vi "Log File Inspector.vi"(1 "Thermocouple types":T4[](array[typedef])=[3, 3, 3, 3, 3, 3, 3, 3, 3, 3, 6, 6, 6, 6, 6, 6] items=["B", "E", "J", "K", "R", "S", "T", "N"], 2 "LC Calibration":T2, 3 "PS Calibration":T3) -> ()   [LabVIEW 2017]
uses:
  Controls/LC Calibration Cluster.ctl
  Support Vis/HOST/cRIO Convert Thermocouple Readings.llb/Thermocouple Type.ctl
  Controls/PS Calibration Cluster.ctl
panel:
  in  "Settings Tab 3":T1(tab)
  out "Temperature Graph":cluster{dbl[], "Y":dbl[]}[](graph)
  out "Pressure Graph":cluster{dbl[], "Y":dbl[]}[](graph)
  out "Load Cell Graph":cluster{dbl[], "Y":dbl[]}[](graph)
  out "Valve Graph":cluster{dbl[], "Y":dbl[]}[](graph)
  in  "Stop Button":bool
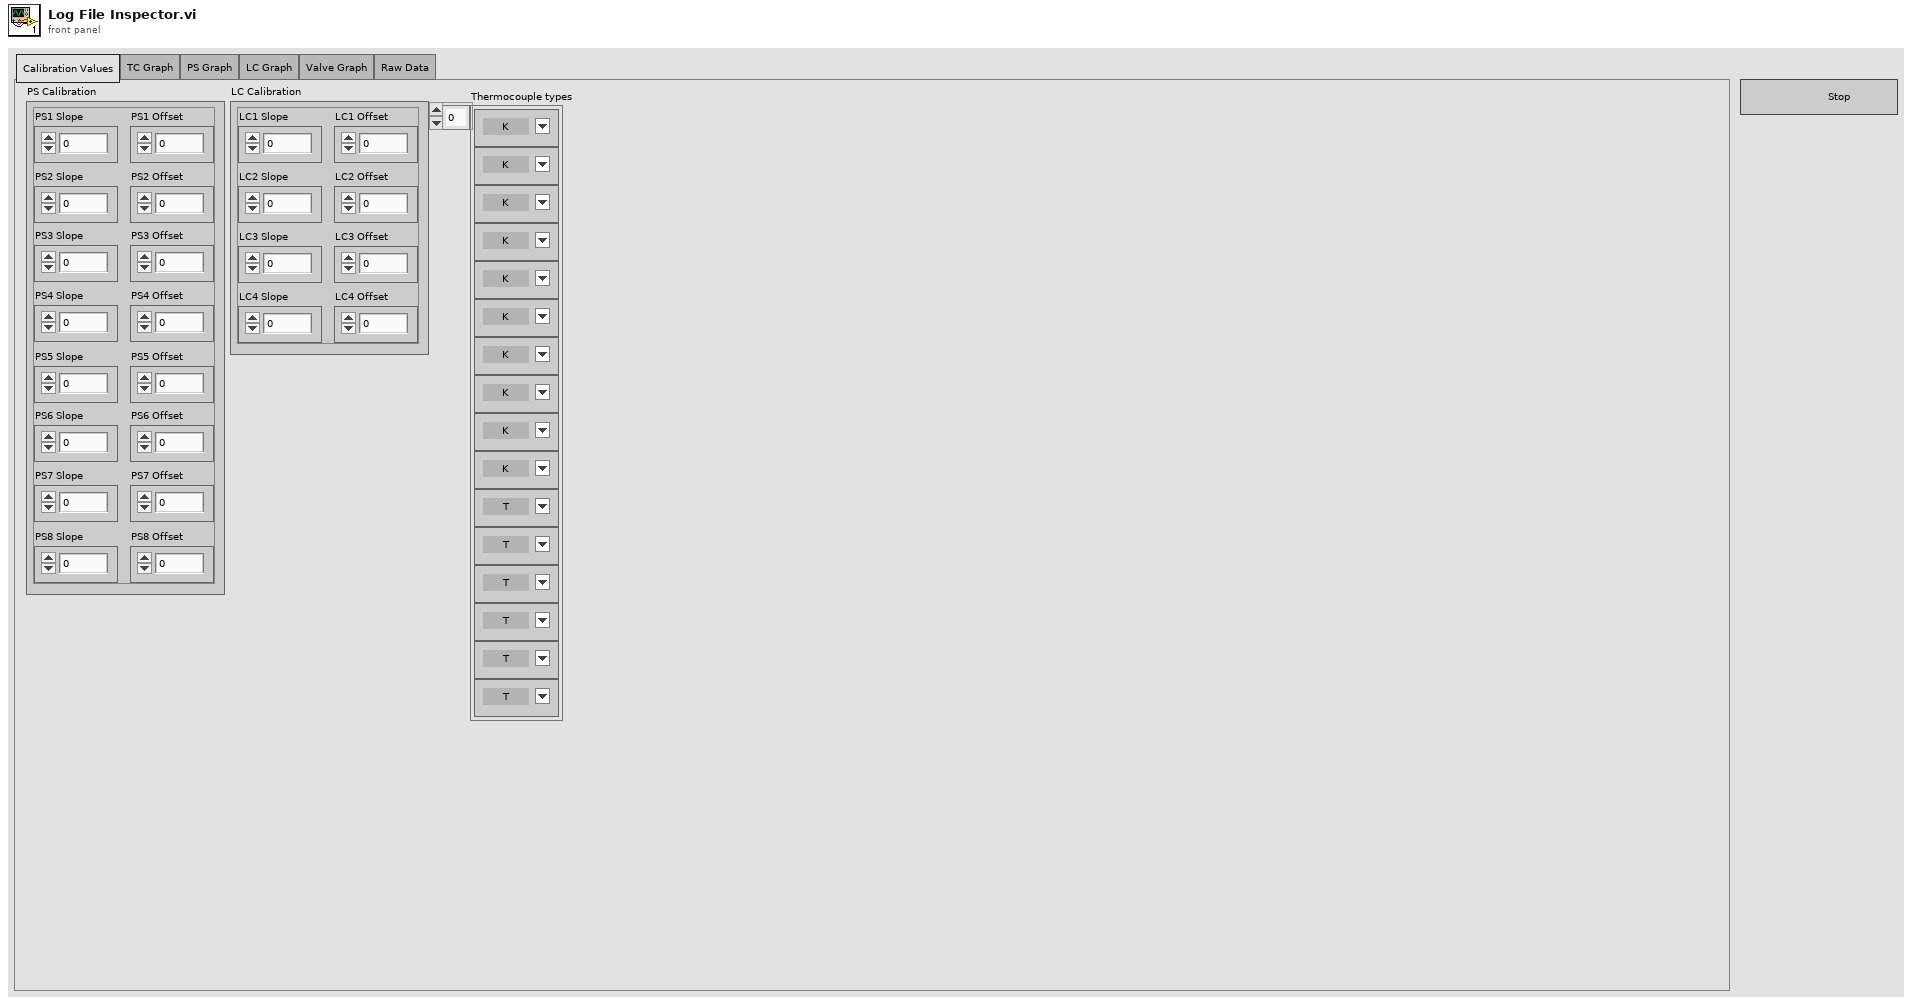
[diagram p1: front panel]
types:
  T1 = enum32{"Calibration Values", "TC Graph", "PS Graph", "LC Graph", "Valve Graph", "Raw Data"}
  T2 = typedef "LC Calibration Cluster.ctl" = cluster{"LC1 Slope":dbl, "LC1 Offset":dbl, "LC2 Slope":dbl, "LC2 Offset":dbl, "LC3 Slope":dbl, "LC3 Offset":dbl, "LC4 Slope":dbl, "LC4 Offset":dbl}
  T3 = typedef "PS Calibration Cluster.ctl" = cluster{"PS1 Slope":dbl, "PS1 Offset":dbl, "PS2 Slope":dbl, "PS2 Offset":dbl, "PS3 Slope":dbl, "PS3 Offset":dbl, "PS4 Slope":dbl, "PS4 Offset":dbl, "PS5 Slope":dbl, "PS5 Offset":dbl, "PS6 Slope":dbl, "PS6 Offset":dbl, "PS7 Slope":dbl, "PS7 Offset":dbl, "PS8 Slope":dbl, "PS8 Offset":dbl}
  T4 = typedef "Thermocouple Type.ctl" = u16
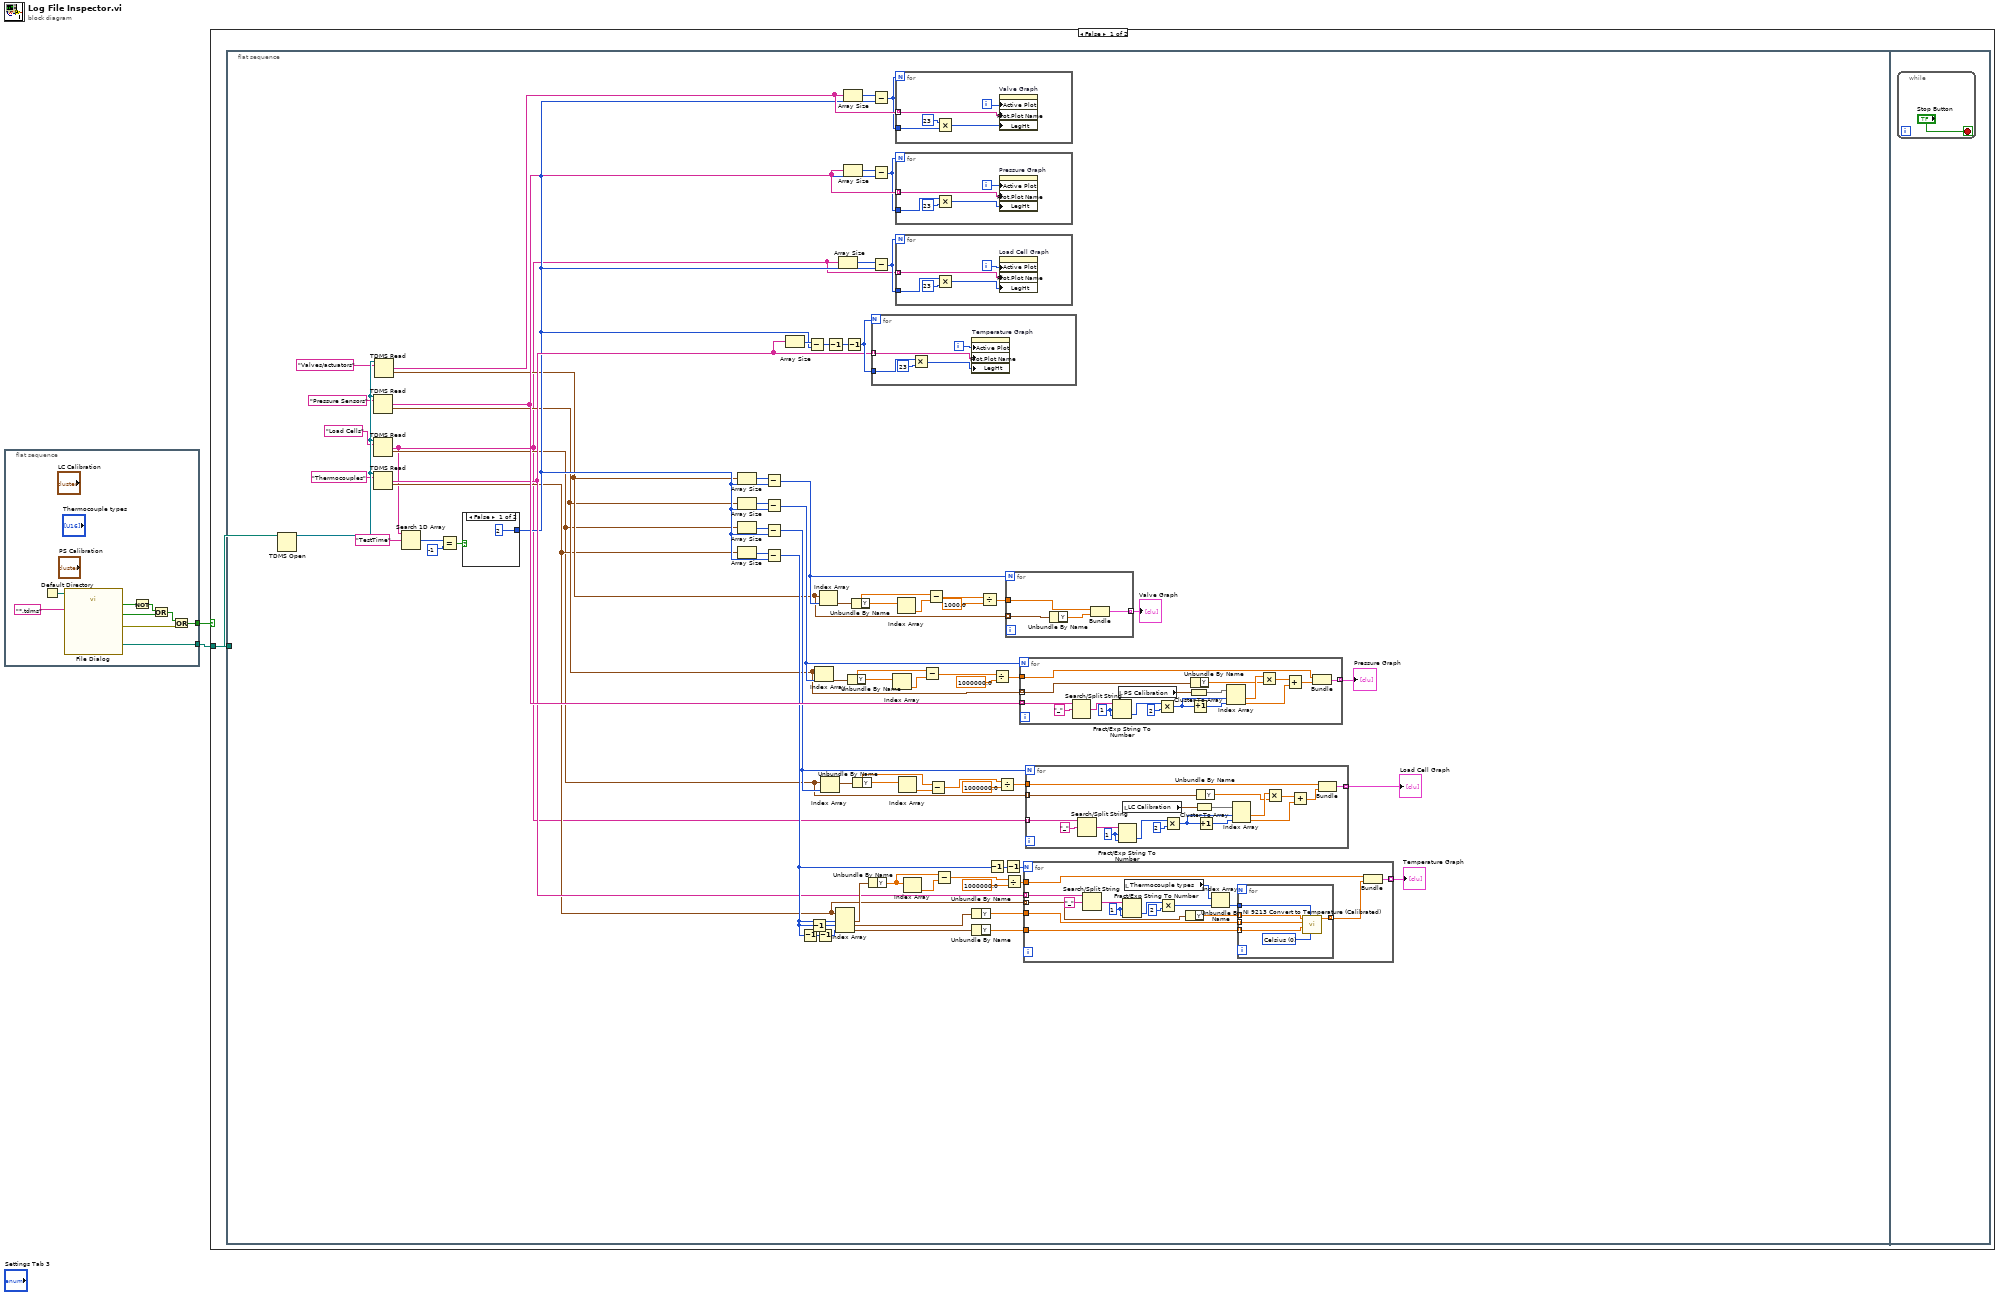
[diagram p0: block diagram]
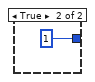
[diagram p2: hidden frame]
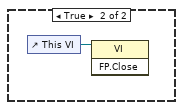
[diagram p3: hidden frame]
diagram:
  n1 = flat-sequence {
    tunnel: [w11] -> w2
    tunnel: [w3] -> w1
    frame #0 {
      n2 = Default Directory() -> (w10:path)
      n3 = call "File Dialog"("start path"=w10, "pattern (all files)"="*.tdms") -> ("selected path"=w11:path, "exists"=w8:bool, "cancelled"=w5:bool, "error out"=w4:errorcluster)  [unwired: 10 in]
      n4 = Not(x=w8) -> (.not. x?=w6:bool)
      n5 = Or(x=w6, y=w5) -> (x .or. y?=w7:bool)
      n6 = Or(x=w7, y=w4) -> (x .or. y?=w3:bool)
    }
  }
  n7 = case shown="False" w1 {
    tunnel: w2 -> [w12 _]
    frame False {
      n8 = flat-sequence {
        tunnel: w12 -> [w84]
        frame #0 {
          n9 = TDMS Open(11:w84) -> (3:w83:refnum<k34>)  [unwired: 6 in, 1 out]
          n10 = TDMS Read(0:w83, 5:"Pressure Sensors" ("group name in")) -> (8:w85:string[], 10:w16:waveform(dbl)[])  [unwired: 6 in, 4 out]
          n11 = TDMS Read(0:w83, 5:"Load Cells" ("group name in")) -> (8:w13:string[], 10:w14:waveform(dbl)[])  [unwired: 6 in, 4 out]
          n12 = TDMS Read(0:w83, 5:"Thermocouples" ("group name in")) -> (8:w19:string[], 10:w15:waveform(dbl)[])  [unwired: 6 in, 4 out]
          n13 = TDMS Read(0:w83, 5:"Valves/actuators" ("group name in")) -> (8:w86:string[], 10:w17:waveform(dbl)[])  [unwired: 6 in, 4 out]
          n14 = Search 1D Array(1D array=w13, element="TestTime") -> (index of element=w81:i32)  [unwired: 1 in]
          n15 = Equal?(x=w81, y=-1) -> (x = y?=w79:bool)
          n16 = case shown="False" w79 {
            tunnel: [2 1] -> w18
            frame False {
            }
            frame True {
            }
          }
          n17 = Array Size(array=w17) -> (size(s)=w66:i32)
          n18 = Array Size(array=w16) -> (size(s)=w50:i32)
          n19 = Array Size(array=w14) -> (size(s)=w41:i32)
          n20 = Array Size(array=w15) -> (size(s)=w59:i32)
          n21 = Subtract(x=w66, y=w18) -> (x-y=w69:i32)
          n22 = Subtract(x=w50, y=w18) -> (x-y=w52:i32)
          n23 = Subtract(x=w41, y=w18) -> (x-y=w43:i32)
          n24 = Subtract(x=w59, y=w18) -> (x-y=w37:i32)
          n25 = Array Size(array=w19) -> (size(s)=w21:i32)
          n26 = Decrement(x=w37) -> (x-1=w34:i32)
          n27 = Subtract(x=w21, y=w18) -> (x-y=w22:i32)
          n28 = Decrement(x=w37) -> (x-1=w36:i32)
          n29 = Index Array(array=w16, index=w52) -> (element=w57:waveform(dbl))
          n30 = Decrement(x=w34) -> (x-1=w35:i32)
          n31 = Index Array(array=w17, index=w69) -> (element=w74:waveform(dbl))
          n32 = Index Array(array=w14, index=w43) -> (element=w48:waveform(dbl))
          n33 = Decrement(x=w22) -> (x-1=w23:i32)
          n34 = Index Array(array=w15, index #1=w37, index #2=w36, index #3=w35) -> (element #1=w65:waveform(dbl), element #2=w33:waveform(dbl), element #3=w32:waveform(dbl))
          n35 = Array Size(array=w13) -> (size(s)=w25:i32)
          n36 = Array Size(array=w86) -> (size(s)=w29:i32)
          n37 = Array Size(array=w85) -> (size(s)=w27:i32)
          n38 = Decrement(x=w23) -> (x-1=w20:i32)
          n39 = Unbundle By Name(w57) -> ("Y"=w56:dbl[])
          n40 = Unbundle By Name(w74) -> ("Y"=w73:dbl[])
          n41 = Unbundle By Name(w48) -> ("Y"=w47:dbl[])
          n42 = Unbundle By Name(w65) -> ("Y"=w64:dbl[])
          n43 = for {
            N: w20 -> [_]
            tunnel: w19 -> [w163] mode=indexing
            tunnel: w20 -> [w159]
            i -> [w162]
            n44 = Multiply(x=w159, y=23) -> (x*y=w161:i32)
            n45 = property on="Temperature Graph" class="XYGraph (strict)"("Active Plot"=w162, "Plot.Plot Name"=w163, "LegHt"=w161) -> ()  [unwired: 2 in, 2 out]
          }
          n46 = Subtract(x=w29, y=w18) -> (x-y=w28:i32)
          n47 = Subtract(x=w27, y=w18) -> (x-y=w26:i32)
          n48 = Subtract(x=w25, y=w18) -> (x-y=w24:i32)
          n49 = Index Array(array=w56) -> (element=w55:dbl)  [unwired: 1 in]
          n50 = for {
            N: w28 -> [_]
            tunnel: w86 -> [w168] mode=indexing
            tunnel: w28 -> [w164]
            i -> [w167]
            n51 = Multiply(x=23, y=w164) -> (x*y=w166:i32)
            n52 = property on="Valve Graph" class="XYGraph (strict)"("Active Plot"=w167, "Plot.Plot Name"=w168, "LegHt"=w166) -> ()  [unwired: 2 in, 2 out]
          }
          n53 = for {
            N: w26 -> [_]
            tunnel: w85 -> [w153] mode=indexing
            tunnel: w26 -> [w149]
            i -> [w152]
            n54 = Multiply(x=w149, y=23) -> (x*y=w151:i32)
            n55 = property on="Pressure Graph" class="XYGraph (strict)"("Active Plot"=w152, "Plot.Plot Name"=w153, "LegHt"=w151) -> ()  [unwired: 2 in, 2 out]
          }
          n56 = for {
            N: w24 -> [_]
            tunnel: w13 -> [w158] mode=indexing
            tunnel: w24 -> [w154]
            i -> [w157]
            n57 = Multiply(x=w154, y=23) -> (x*y=w156:i32)
            n58 = property on="Load Cell Graph" class="XYGraph (strict)"("Active Plot"=w157, "Plot.Plot Name"=w158, "LegHt"=w156) -> ()  [unwired: 2 in, 2 out]
          }
          n59 = Index Array(array=w73) -> (element=w72:dbl)  [unwired: 1 in]
          n60 = Index Array(array=w47) -> (element=w46:dbl)  [unwired: 1 in]
          n61 = Index Array(array=w64) -> (element=w63:dbl)  [unwired: 1 in]
          n62 = Subtract(x=w56, y=w55) -> (x-y=w53:dbl[])
          n63 = Subtract(x=w73, y=w72) -> (x-y=w70:dbl[])
          n64 = Subtract(x=w47, y=w46) -> (x-y=w44:dbl[])
          n65 = Subtract(x=w64, y=w63) -> (x-y=w61:dbl[])
          n66 = Unbundle By Name(w33) -> ("Y"=w31:dbl[])
          n67 = Unbundle By Name(w32) -> ("Y"=w30:dbl[])
          n68 = Divide(x=w70, y=1000.0) -> (x/y=w68:dbl[])
          n69 = Decrement(x=w37) -> (x-1=w39:i32)
          n70 = Divide(x=w53, y=1000000.0) -> (x/y=w51:dbl[])
          n71 = Divide(x=w44, y=1000000.0) -> (x/y=w42:dbl[])
          n72 = Decrement(x=w39) -> (x-1=w38:i32)
          n73 = Divide(x=w61, y=1000000.0) -> (x/y=w60:dbl[])
          n74 = for {
            N: w69 -> [_]
            tunnel: w17 -> [w148] mode=indexing
            tunnel: [w146] -> w67 mode=indexing
            tunnel: w68 -> [w145]
            n75 = Unbundle By Name(w148) -> ("Y"=w147:dbl[])
            n76 = Bundle(w145, "Y"=w147) -> (w146:cluster{dbl[], "Y":dbl[]})  [unwired: 1 in]
          }
          "Valve Graph" <- w67
          n77 = for {
            N: w52 -> [_]
            tunnel: w16 -> [w122] mode=indexing
            tunnel: [w121] -> w49 mode=indexing
            tunnel: w51 -> [w120]
            tunnel: w85 -> [w114] mode=indexing
            w118 = 1
            n78 = Search/Split String(string=w114, search string/char (-)="_") -> (match + rest of string=w117:string)  [unwired: 1 in, 2 out]
            n79 = Fract/Exp String To Number(string=w117, offset=w118, default (0 dbl)=w118) -> (number=w115:i32)  [unwired: 1 in, 1 out]
            n80 = local read "PS Calibration"() -> (w113:T3)
            n81 = Multiply(x=w115, y=2 ("number")) -> (x*y=w111:i32)
            n82 = Cluster To Array(cluster=w113) -> (array=w112:dbl[])
            n83 = Unbundle By Name(w122) -> ("Y"=w108:dbl[])
            n84 = Increment(x=w111) -> (x+1=w110:i32)
            n85 = Index Array(array=w112, index #1=w111, index #2=w110) -> (element #1=w109:dbl, element #2=w107:dbl)
            n86 = Multiply(x=w109, y=w108) -> (x*y=w106:dbl[])
            n87 = Add(x=w106, y=w107) -> (x+y=w105:dbl[])
            n88 = Bundle(w120, w105) -> (w121:cluster{dbl[], dbl[]})  [unwired: 1 in]
          }
          "Pressure Graph" <- w49
          n89 = for {
            N: w38 -> [_]
            tunnel: w15 -> [w131] mode=indexing
            tunnel: [w123] -> w58 mode=indexing
            tunnel: w60 -> [w130]
            tunnel: w19 -> [w132] mode=indexing
            tunnel: w31 -> [w126]
            tunnel: w30 -> [w125]
            w137 = 1
            n90 = Search/Split String(string=w132, search string/char (-)="_") -> (match + rest of string=w136:string)  [unwired: 1 in, 2 out]
            n91 = Fract/Exp String To Number(string=w136, offset=w137, default (0 dbl)=w137) -> (number=w134:i32)  [unwired: 1 in, 1 out]
            n92 = local read "Thermocouple types"() -> (w127:T4[])
            n93 = Multiply(x=w134, y=2 ("number")) -> (x*y=w133:i32)
            n94 = Unbundle By Name(w131) -> ("Y"=w129:dbl[])
            n95 = Index Array(array=w127, index=w133) -> (element=w128:T4)
            n96 = for {
              tunnel: w129 -> [w142] mode=indexing
              tunnel: w128 -> [w139]
              tunnel: w126 -> [w144] mode=indexing
              tunnel: w125 -> [w143] mode=indexing
              tunnel: [w140] -> w124 mode=indexing
              w141 = u16 0 items=["Celsius", "Fahrenheit", "Kelvin", "Rankine"] ("Temperature Units (C)")
              n97 = call "NI 9213 Convert to Temperature (Calibrated).vi"("Temperature Units (C)"=w141, "ThermocoupleType"=w139, "AutoZero"=w143, "CJC"=w144, "TC Input"=w142) -> ("Thermocouple Temperature"=w140:dbl)  [unwired: 6 in]
            }
            n98 = Bundle(w130, w124) -> (w123:cluster{dbl[], dbl[]})  [unwired: 1 in]
          }
          "Temperature Graph" <- w58
          n99 = for {
            N: w43 -> [_]
            tunnel: w14 -> [w91] mode=indexing
            tunnel: [w92] -> w40 mode=indexing
            tunnel: w42 -> [w89]
            tunnel: w13 -> [w90] mode=indexing
            w103 = 1
            n100 = Search/Split String(string=w90, search string/char (-)="_") -> (match + rest of string=w102:string)  [unwired: 1 in, 2 out]
            n101 = Fract/Exp String To Number(string=w102, offset=w103, default (0 dbl)=w103) -> (number=w100:i32)  [unwired: 1 in, 1 out]
            n102 = local read "LC Calibration"() -> (w88:T2)
            n103 = Multiply(x=w100, y=2 ("number")) -> (x*y=w99:i32)
            n104 = Cluster To Array(cluster=w88) -> (array=w87:dbl[])
            n105 = Unbundle By Name(w91) -> ("Y"=w96:dbl[])
            n106 = Increment(x=w99) -> (x+1=w98:i32)
            n107 = Index Array(array=w87, index #1=w99, index #2=w98) -> (element #1=w97:dbl, element #2=w95:dbl)
            n108 = Multiply(x=w97, y=w96) -> (x*y=w94:dbl[])
            n109 = Add(x=w94, y=w95) -> (x+y=w93:dbl[])
            n110 = Bundle(w89, w93) -> (w92:cluster{dbl[], dbl[]})  [unwired: 1 in]
          }
          "Load Cell Graph" <- w40
        }
        frame #1 {
          n111 = while {
            stop <- "Stop Button" stop-if-true
          }
        }
      }
    }
    frame True {
      n112 = control-ref of="This VI"() -> (w172:refnum<vi>)
      n113 = invoke class="VI" method="FP.Close"(reference=w172) -> ()  [unwired: 2 in, 3 out]
    }
  }
